vi "Initialize.vi"(8 "error in":errorcluster) -> (0 "error out":errorcluster, 2 "Readiness Check Results":T1[](array[typedef]), 3 "Framework Engine":refnum<class "Framework Engine.lvclass">)   [LabVIEW 2026, in "Framework Engine.lvclass"]
uses:
  Framework Engine.lvclass
  Framework Engine.lvclass/Framework Engine.ctl
  Services/Settings Service/Settings Service.lvclass
  Services/Logging Service/Logging Service.lvclass
  Services/Readiness Service/Readines Service.lvclass
  Typedefs/enums/Readiness State Enum.ctl
  Typedefs/clusters/Readiness Check Result.ctl
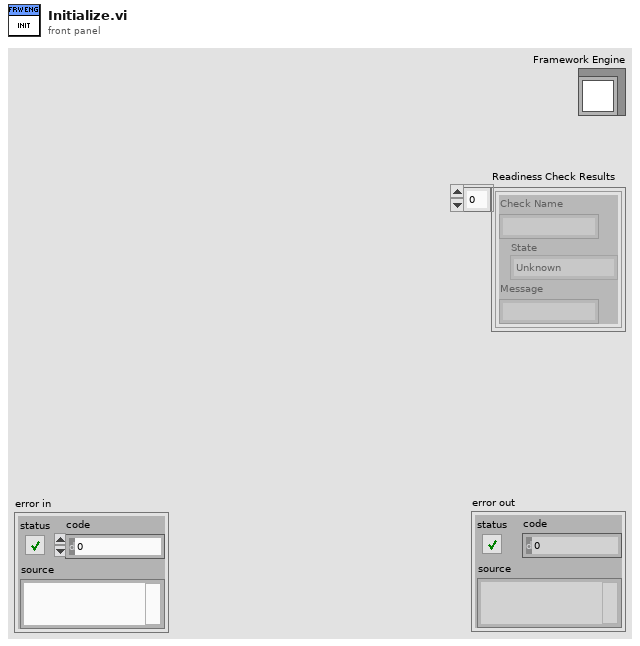
[diagram p1: front panel]
types:
  T1 = typedef "Readiness Check Result.ctl" = cluster{"Check Name":string, "State":T2, "Message":string}
  T2 = typedef "Readiness State Enum.ctl" = enum16{"Unknown", "Ready", "Warning", "NotReady"}
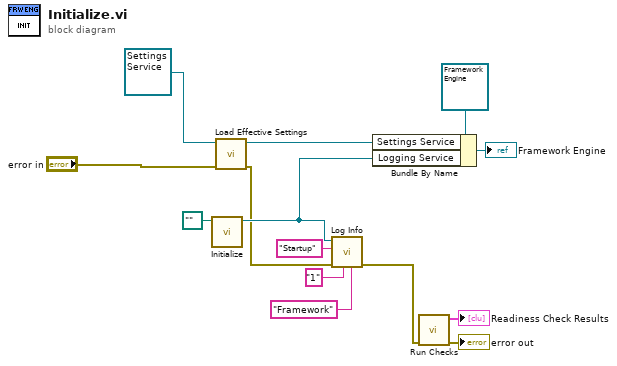
[diagram p0: block diagram]
diagram:
  n1 = call "Initialize.vi"("Log File Path"=path "") -> ("Data"=w10:refnum<class "Logging Service.lvclass">)  [unwired: 10 in]
  n2 = call "Load Effective Settings.vi"("error in"="error in", "Settings Service in"=refnum<class "Settings Service.lvclass"> refnum) -> ("error out"=w8:errorcluster, "Setting Service out"=w13:refnum<class "Settings Service.lvclass">)  [unwired: 8 in]
  n3 = call "Log Info.vi"("User"="Framework", "Level"="1", "error in"=w8, "Message"="Startup", "Data"=w10) -> ("error out"=w4:errorcluster)  [unwired: 6 in]
  n4 = Bundle By Name(cluster=refnum<class "Framework Engine.lvclass"> refnum ("Framework Engine.lvclass"), "Settings Service"=w13, "Logging Service"=w10) -> (→"Framework Engine":refnum<class "Framework Engine.lvclass">)
  n5 = call "Run Checks.vi"("error in (no error)"=w4) -> ("error out"=→"error out":errorcluster, "Readiness Check Results"=→"Readiness Check Results":T1[])  [unwired: 9 in]
